vi "Find Mirror.vi"(11 "Array in":string[][](array[string])) -> (1 "set":set{i32}(c389), 2 "element":i32, 3 "Array out":i32[](array[numeric]))   [LabVIEW 2021]
uses:
  fea15efd-061a-4aee-a98b-c59d17ea33de.vi
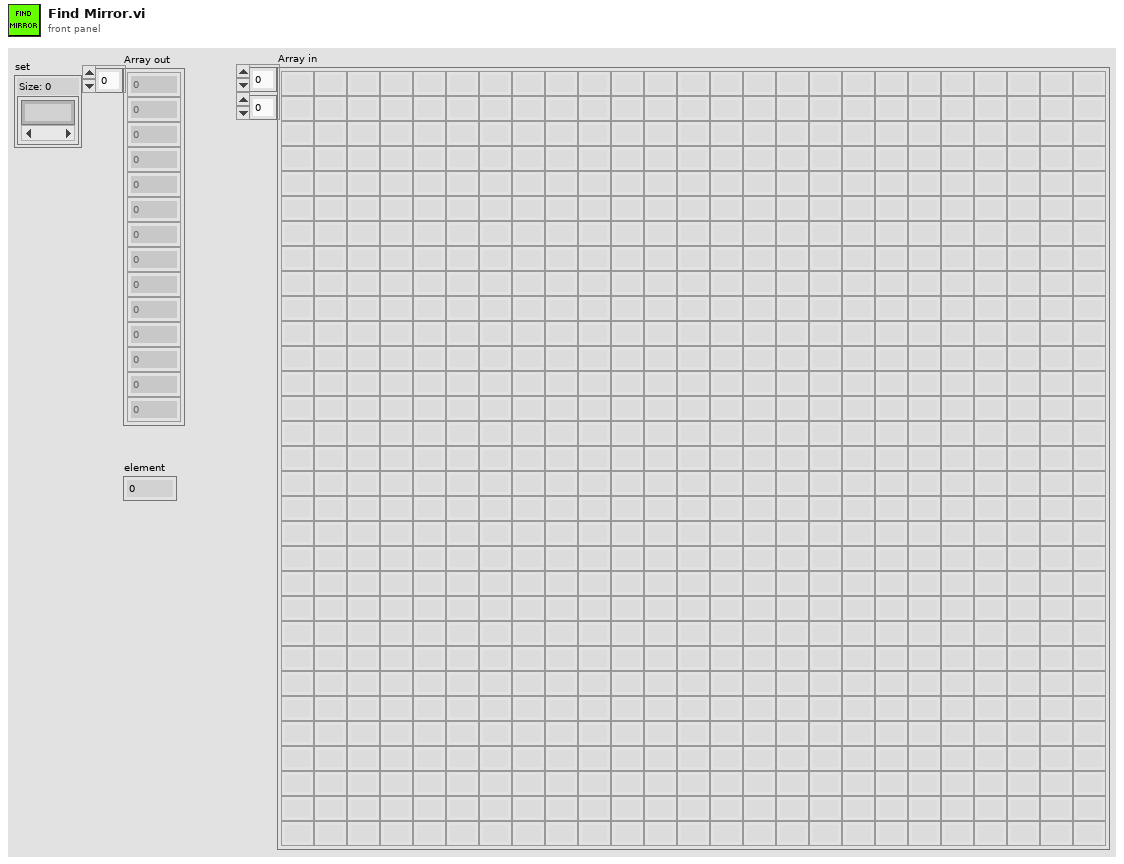
[diagram p1: front panel]
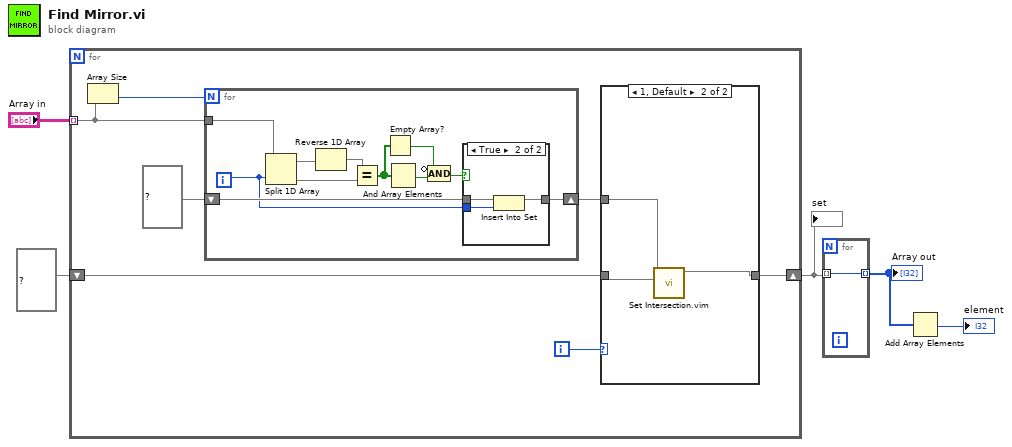
[diagram p0: block diagram]
diagram:
  n1 = for {
    tunnel: "Array in" -> [w11] mode=indexing
    shift-right: [w8] -> w1
    shift-left: set{i32} {} ("set") -> [w6]
    i -> [w9]
    n2 = Array Size(array=w11) -> (size(s)=w12:i32)
    n3 = for {
      N: w12 -> [_]
      tunnel: w11 -> [w27]
      shift-right: [w22] -> w7
      shift-left: set{i32} {} ("set") -> [w23]
      i -> [w21]
      n4 = Split 1D Array(array=w27, index=w21) -> (first subarray=w26:string[], second subarray=w24:string[])
      n5 = Reverse 1D Array(array=w26) -> (reversed array=w25:string[])
      n6 = Equal?(x=w25, y=w24) -> (x = y?=w20:bool[])
      n7 = Empty Array?(array=w20) -> (empty?=w17:bool)
      n8 = And Array Elements(Boolean array=w20) -> (logical AND=w18:bool)
      n9 = Compound Arithmetic op=AND(invert w17, w18) -> (w19:bool)
      n10 = case shown="True" w19 {
        tunnel: w23 -> [w28 w31]
        tunnel: [w28 w30] -> w22
        tunnel: w21 -> [_ w29]
        frame False {
        }
        frame True {
          n11 = Insert Into Set(10:w29, 11:w31) -> (3:w30:set{i32})  [unwired: 1 out]
        }
      }
    }
    n12 = case shown="1, Default" w9 {
      tunnel: [w13 w14] -> w8
      tunnel: w7 -> [w13 w15]
      tunnel: w6 -> [_ w16]
      frame 0 {
      }
      frame 1, Default {
        n13 = call "Set Intersection.vim"("set 2"=w16, "set 1"=w15) -> ("intersection"=w14:set{i32})  [unwired: 9 in]
      }
    }
  }
  "set" <- w1
  n14 = for {
    tunnel: [w32] -> w2 mode=indexing
    tunnel: w1 -> [w32] mode=indexing
  }
  "Array out" <- w2
  n15 = Add Array Elements(numeric array=w2) -> (sum=→"element":i32)
